vi "rs3 delete device list.vi"(8 "error in (no error)":errorcluster, 11 "device list":u64) -> (0 "error out":errorcluster)   [LabVIEW 2017, in "libRealSense3.lvlib"]
doc: "Delete the device list after all devices have been deleted."
uses:
  libRealSense3.lvlib
  realsense2.dll
panel:
  # "RS3 Delete Device List"
  # "(C) Intel Corp. 2017,  AGJ"
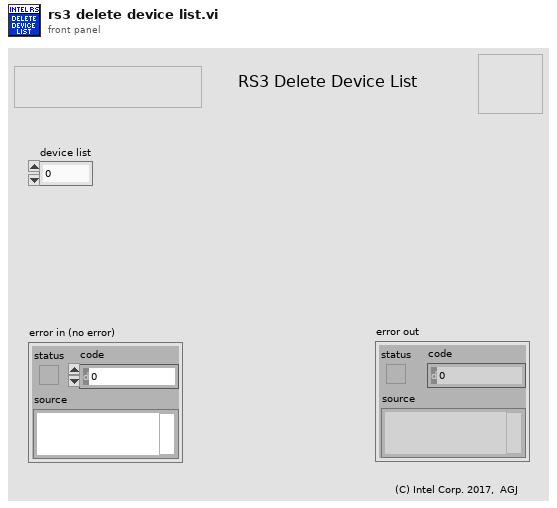
[diagram p1: front panel]
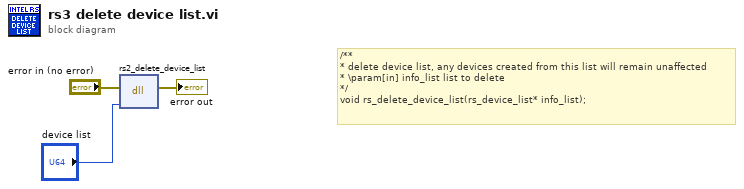
[diagram p0: block diagram]
diagram:
  # "/**\n* delete device list, any devices created from this list will remain unaffected\n* \\param[in] info_list list to delete\n*/\nvoid rs_delete_device_list(rs_device_list* info_list);"
  n1 = dll-call lib="C:/Users/smartek/Desktop/labview/realsense2.dll" fn="rs2_delete_device_list"(error in="error in (no error)", "device list"="device list") -> (error out=→"error out":errorcluster)  [unwired: 4 in, 1 out]
